vi "run_ending_set_v02.vi"(8 "error in":errorcluster, 9 "data in":T1={"daq_ao 1"="Dev1/ao0", "daq_ai 1"="Dev1/ai0", "experiment day folder"=path "D:/DATA/8-27-15 save func testing/test.lvm", "Multiclamp init error"=0, "Multiclamp Handle Out"=0, "sampling rate (Hz)"=10000, "trial name"=""}, 11 "controls array in":refnum<vi>[](array[refnum])) -> (0 "error out":errorcluster, 1 "data out":T1={"daq_ao 1"="Dev1/ao0", "daq_ai 1"="Dev1/ai0", "experiment day folder"=path "D:/DATA/8-27-15 save func testing/test.lvm", "Multiclamp init error"=0, "Multiclamp Handle Out"=0, "sampling rate (Hz)"=10000, "trial name"=""}, 3 "control array out":refnum<vi>[](array[refnum]))   [LabVIEW 2015]
uses:
  get_data_from_control_tfarray.vi
  Controls/Data.ctl
panel:
  out "ENDING TF set":T2
  # "RUN ENDING SET AUTO WC"
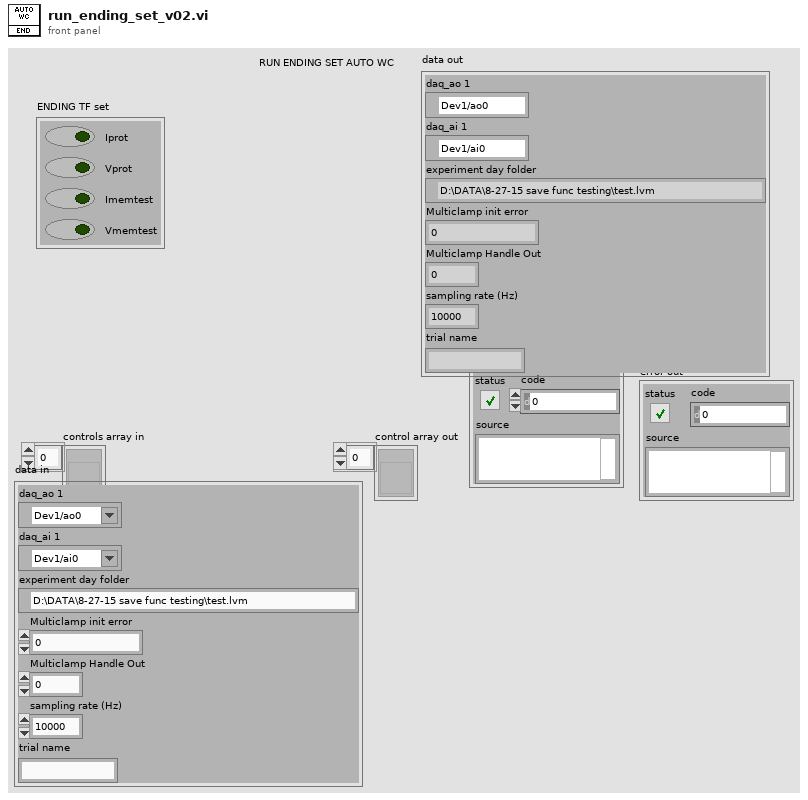
[diagram p1: front panel]
types:
  T1 = typedef "Data.ctl" = cluster{"daq_ao 1":tag, "daq_ai 1":tag, "experiment day folder":path, "Multiclamp init error":i32, "Multiclamp Handle Out":u32, "sampling rate (Hz)":i32, "trial name":string}
  T2 = cluster{" Iprot":bool, " Vprot":bool, " Imemtest":bool, " Vmemtest":bool}
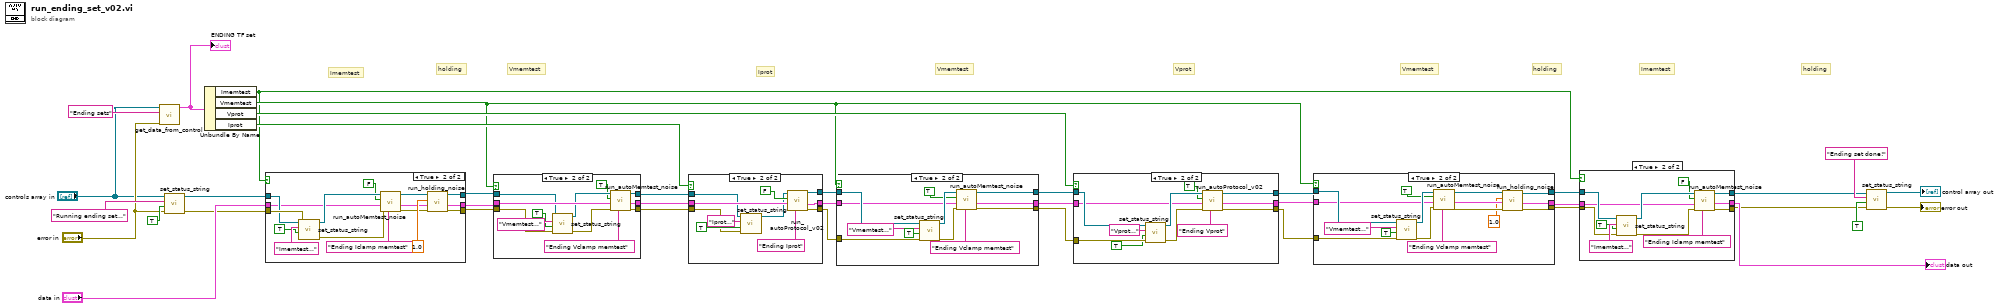
[diagram p0: block diagram]
diagram:
  # "Imemtest"
  # "Vmemtest"
  # "Vmemtest"
  # "holding"
  # "Vmemtest"
  # "holding"
  # "holding"
  # "Imemtest"
  # "Vprot"
  # "Iprot"
  n1 = call-poly "get_data_from_control.vi"("error in"="error in", "control label"="Ending sets", "controls array"="controls array in") -> ("TF set out"=w38:T2)  [unwired: 7 in, 1 out]
  "ENDING TF set" <- w38
  n2 = call "set_status_string.vi"("error in"="error in", "new line?"=TRUE, "status string in"="Running ending set...", "controls array"="controls array in") -> ("error out"=w1:errorcluster, "controls array out"=w2:refnum<vi>[])  [unwired: 6 in]
  n3 = Unbundle By Name(w38) -> ("Imemtest"=w16:bool, "Vmemtest"=w17:bool, "Vprot"=w24:bool, "Iprot"=w37:bool)
  n4 = case shown="True" w16 {
    tunnel: [w41 w42] -> w12
    tunnel: [w39 w44] -> w10
    tunnel: [w40 w43] -> w11
    tunnel: w1 -> [w39 w51]
    tunnel: w2 -> [w41 w50]
    tunnel: "data in" -> [w40 w49]
    frame False {
    }
    frame True {
      n5 = call "set_status_string.vi"("error in"=w51, "new line?"=TRUE, "status string in"="Imemtest...", "controls array"=w50) -> ("error out"=w53:errorcluster, "controls array out"=w56:refnum<vi>[])  [unwired: 6 in]
      n6 = call "run_autoMemtest_noise.vi"("control label"="Ending Iclamp memtest", "error in"=w53, "data in"=w49, "clamp switch (T=v, F=i)"=FALSE, "controls array"=w56) -> ("error out"=w46:errorcluster, "data out"=w45:T1, "controls out"=w47:refnum<vi>[])  [unwired: 2 in, 2 out]
      n7 = call "run_holding_noise.vi"("error in"=w46, "data in"=w45, "holding time (s)"=1.0, "controls array in"=w47) -> ("error out"=w44:errorcluster, "data out"=w43:T1, "controls array out"=w42:refnum<vi>[])  [unwired: 4 in, 1 out]
    }
  }
  n8 = case shown="True" w17 {
    tunnel: w12 -> [w60 w71]
    tunnel: w10 -> [w58 w67]
    tunnel: w11 -> [w59 w72]
    tunnel: [w60 w65] -> w33
    tunnel: [w59 w64] -> w32
    tunnel: [w58 w63] -> w31
    frame False {
    }
    frame True {
      n9 = call "set_status_string.vi"("error in"=w67, "new line?"=TRUE, "status string in"="Vmemtest...", "controls array"=w71) -> ("error out"=w66:errorcluster, "controls array out"=w70:refnum<vi>[])  [unwired: 6 in]
      n10 = call "run_autoMemtest_noise.vi"("control label"="Ending Vclamp memtest", "error in"=w66, "data in"=w72, "clamp switch (T=v, F=i)"=TRUE, "controls array"=w70) -> ("error out"=w63:errorcluster, "data out"=w64:T1, "controls out"=w65:refnum<vi>[])  [unwired: 2 in, 2 out]
    }
  }
  n11 = case shown="True" w37 {
    tunnel: w33 -> [w75 w80]
    tunnel: w32 -> [w73 w83]
    tunnel: w31 -> [w74 w84]
    tunnel: [w75 w78] -> w27
    tunnel: [w74 w77] -> w26
    tunnel: [w73 w76] -> w25
    frame False {
    }
    frame True {
      n12 = call "set_status_string.vi"("error in"=w84, "new line?"=TRUE, "status string in"="Iprot...", "controls array"=w80) -> ("controls array out"=w79:refnum<vi>[])  [unwired: 6 in, 1 out]
      n13 = call "run_autoProtocol_v02.vi"("control label"="Ending Iprot", "data in"=w83, "clamp switch (T=v, F=i)"=FALSE, "controls array"=w79) -> ("error out"=w77:errorcluster, "data out"=w76:T1, "controls array out"=w78:refnum<vi>[])  [unwired: 5 in]
    }
  }
  n14 = case shown="True" w17 {
    tunnel: w27 -> [w89 w101]
    tunnel: w26 -> [w87 w99]
    tunnel: w25 -> [w88 w96]
    tunnel: [w89 w92] -> w23
    tunnel: [w87 w91] -> w22
    tunnel: [w88 w90] -> w21
    frame False {
    }
    frame True {
      n15 = call "set_status_string.vi"("error in"=w99, "new line?"=TRUE, "status string in"="Vmemtest...", "controls array"=w101) -> ("error out"=w98:errorcluster, "controls array out"=w100:refnum<vi>[])  [unwired: 6 in]
      n16 = call "run_autoMemtest_noise.vi"("control label"="Ending Vclamp memtest", "error in"=w98, "data in"=w96, "clamp switch (T=v, F=i)"=TRUE, "controls array"=w100) -> ("error out"=w91:errorcluster, "data out"=w90:T1, "controls out"=w92:refnum<vi>[])  [unwired: 2 in, 2 out]
    }
  }
  n17 = case shown="True" w24 {
    tunnel: w23 -> [w104 w116]
    tunnel: w22 -> [w102 w115]
    tunnel: w21 -> [w103 w109]
    tunnel: [w104 w107] -> w20
    tunnel: [w103 w106] -> w19
    tunnel: [w102 w105] -> w18
    frame False {
    }
    frame True {
      n18 = call "set_status_string.vi"("error in"=w115, "new line?"=TRUE, "status string in"="Vprot...", "controls array"=w116) -> ("error out"=w112:errorcluster, "controls array out"=w113:refnum<vi>[])  [unwired: 6 in]
      n19 = call "run_autoProtocol_v02.vi"("control label"="Ending Vprot", "error in"=w112, "data in"=w109, "clamp switch (T=v, F=i)"=TRUE, "controls array"=w113) -> ("error out"=w105:errorcluster, "data out"=w106:T1, "controls array out"=w107:refnum<vi>[])  [unwired: 4 in]
    }
  }
  n20 = case shown="True" w17 {
    tunnel: w20 -> [w119 w135]
    tunnel: w18 -> [w117 w133]
    tunnel: w19 -> [w118 w130]
    tunnel: [w119 w123] -> w9
    tunnel: [w117 w121] -> w7
    tunnel: [w118 w122] -> w8
    frame False {
    }
    frame True {
      n21 = call "set_status_string.vi"("error in"=w133, "new line?"=TRUE, "status string in"="Vmemtest...", "controls array"=w135) -> ("error out"=w132:errorcluster, "controls array out"=w134:refnum<vi>[])  [unwired: 6 in]
      n22 = call "run_autoMemtest_noise.vi"("control label"="Ending Vclamp memtest", "error in"=w132, "data in"=w130, "clamp switch (T=v, F=i)"=TRUE, "controls array"=w134) -> ("error out"=w125:errorcluster, "data out"=w124:T1, "controls out"=w126:refnum<vi>[])  [unwired: 2 in, 2 out]
      n23 = call "run_holding_noise.vi"("error in"=w125, "data in"=w124, "holding time (s)"=1.0, "controls array in"=w126) -> ("error out"=w121:errorcluster, "data out"=w122:T1, "controls array out"=w123:refnum<vi>[])  [unwired: 4 in, 1 out]
    }
  }
  n24 = case shown="True" w16 {
    tunnel: w9 -> [w138 w150]
    tunnel: w7 -> [w137 w142]
    tunnel: [w138 w146] -> w6
    tunnel: [w137 w145] -> w4
    tunnel: [w136 w144] -> w5
    tunnel: w8 -> [w136 w139]
    frame False {
    }
    frame True {
      n25 = call "set_status_string.vi"("error in"=w142, "new line?"=TRUE, "status string in"="Imemtest...", "controls array"=w150) -> ("error out"=w141:errorcluster, "controls array out"=w148:refnum<vi>[])  [unwired: 6 in]
      n26 = call "run_autoMemtest_noise.vi"("control label"="Ending Iclamp memtest", "error in"=w141, "data in"=w139, "clamp switch (T=v, F=i)"=FALSE, "controls array"=w148) -> ("error out"=w145:errorcluster, "data out"=w144:T1, "controls out"=w146:refnum<vi>[])  [unwired: 2 in, 2 out]
    }
  }
  "data out" <- w5
  n27 = call "set_status_string.vi"("error in"=w4, "new line?"=TRUE, "status string in"="Ending set done!", "controls array"=w6) -> ("error out"=→"error out":errorcluster, "controls array out"=→"control array out":refnum<vi>[])  [unwired: 6 in]
